vi "GetPitchValuesINI.vi"(8 "error in (no error)":errorcluster, 11 "configuration file path":path) -> (0 "error out":errorcluster, 1 "PitchFiring":dbl, 2 "PitchLoading":dbl, 3 "file path":path, 4 "PitchMax":dbl, 6 "PitchMin":dbl)   [LabVIEW 2012]
uses:
  <vilib>/Utility/config.llb/Read Key (Double).vi
  <vilib>/Utility/config.llb/NI_LVConfig.lvlib
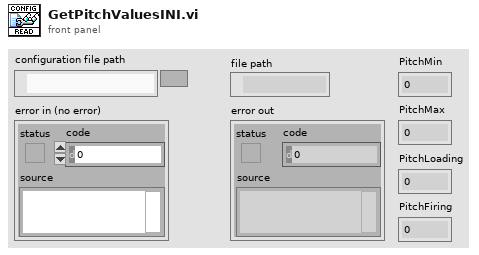
[diagram p1: front panel]
types:
  T1 = typedef "NI_LVConfig.lvlib/Config Data RefNum.ctl" = refnum<k1>
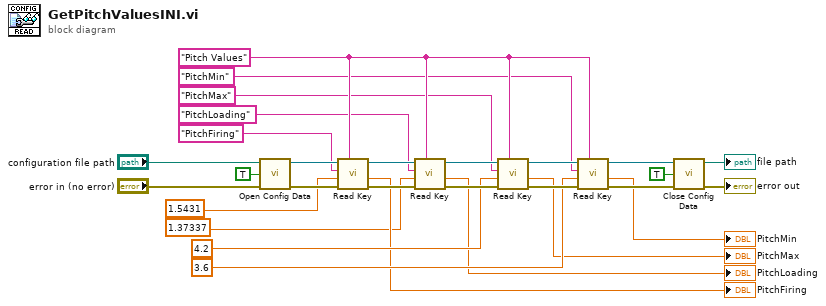
[diagram p0: block diagram]
diagram:
  w7 = "Pitch Values"
  n1 = call <vilib>:"Open Config Data.vi"("error in (no error)"="error in (no error)", "create file if necessary (T)"=TRUE, "configuration file path"="configuration file path") -> ("error out"=w25:errorcluster, "refnum"=w26:T1)  [unwired: 6 in, 1 out]
  n2 = call-poly <vilib>:"Read Key.vi"("section"=w7, "error in (no error)"=w25, "default value"=1.5431, "key"="PitchFiring", "refnum"=w26) -> ("error out"=w23:errorcluster, "value"=→"PitchFiring":dbl, "refnum out"=w24:T1)  [unwired: 3 in, 1 out]
  n3 = call-poly <vilib>:"Read Key.vi"("section"=w7, "error in (no error)"=w23, "default value"=1.37337, "key"="PitchLoading", "refnum"=w24) -> ("error out"=w29:errorcluster, "value"=→"PitchLoading":dbl, "refnum out"=w14:T1)  [unwired: 3 in, 1 out]
  n4 = call-poly <vilib>:"Read Key.vi"("section"=w7, "error in (no error)"=w29, "default value"=4.2, "key"="PitchMax", "refnum"=w14) -> ("error out"=w17:errorcluster, "value"=→"PitchMax":dbl, "refnum out"=w18:T1)  [unwired: 3 in, 1 out]
  n5 = call-poly <vilib>:"Read Key.vi"("section"=w7, "error in (no error)"=w17, "default value"=3.6, "key"="PitchMin", "refnum"=w18) -> ("error out"=w16:errorcluster, "value"=→"PitchMin":dbl, "refnum out"=w15:T1)  [unwired: 3 in, 1 out]
  n6 = call <vilib>:"Close Config Data.vi"("error in (no error)"=w16, "write file if changed (T)"=TRUE, "refnum"=w15) -> ("error out"=→"error out":errorcluster, "file path"=→"file path":path)  [unwired: 7 in]
